vi "PDC_Port.vi"() -> ()   [LabVIEW 2011]
uses:
  <vilib>/Utility/tcp.llb/UDP Multicast Write-Only Open.vi
  <vilib>/Utility/xml.llb/Write to XML File(string).vi
  <vilib>/Utility/xml.llb/Read From XML File(array).vi
  Windows/System32/user32.dll
panel:
  out "output array 5":string[](array[string])
  in  "Analog Params":string[](array[string])
  out "user event out":refnum<user-event>
  in  "Tab Control 3":T1(tab)
  out "Phasor Name":string[](array[string])
  out "Complex Format":cdb[](array[numeric])
  in  "?":i32(listbox)
  out "?":i32(listbox)
  out "?":i32[](listbox)
  out "index of element":i32
  in  "A2":bool[](array[boolean])
  in  "Phasor   Angle":string[](array[string])
  in  "Phasor    Amplitude":string[](array[string])
  out "Row2":i32
  in  "A1":bool[](array[boolean])
  in  "Img":dbl[](array[numeric])
  in  "Real":dbl[](array[numeric])
  in  "Analog Parameters":i32(listbox)
  in  "Digital Parameters":i32(listbox)
  out "Complex":cdb[](array[numeric])
  out "element 2":string
  out "Digital Signal Indicator":bool[][](array[boolean])
  in  "Digital Params":string[](array[string])
  out "element 3":string
  out "Analog Size":i32
  out "Digital Size":i32
  in  "output array":string[](array[string])
  in  "Phasor Item502":string
  in  "Phasor Item402":string
  in  "Phasor Item302":string
  in  "Phasor Item202":string
  in  "Phasor Item102":string
  in  "Phasor Item44":string
  in  "Phasor Item34":string
  in  "Phasor Item24":string
  in  "Phasor Item14":string
  in  "Phasor Item43":string
  in  "Phasor Item33":string
  in  "Phasor Item23":string
  in  "Phasor Item13":string
  in  "Phasor Item42":string
  in  "Phasor Item32":string
  in  "Phasor Item22":string
  in  "Phasor Item12":string
  in  "Phasor Item4":string
  in  "Phasor Item3":string
  in  "Phasor Item2":string
  in  "Phasor Item1":string
  in  "Tab Control 2":T2(tab)
  out "Quitting 2":bool
  in  "Quit 2":bool
  in  "Digital String":string[](array[string])
  in  "Digital Signal":dbl[](array[numeric])
  in  "DFREQ Values":dbl[](array[numeric])
  in  "FREQ Values":dbl[](array[numeric])
  in  "Phasor Values":dbl[](array[numeric])
  in  "Phasor Time":string[](array[string])
  in  "Play Chosen Data":bool
  in  "Load Configuration":bool
  in  "Save Configuration":bool
  out "?":i32[](listbox)
  in  "MA":string
  out "Row of phasor parameter":i32
  out "initialized array":string[](array[string])
  in  "Analog Signal":dbl[](array[numeric])
  out "XML Open File Path":path=path "C:/Users/iitc1/Documents"
  out "XML File Save Path":path
  out "Phasor Index":i32[](array[numeric])
  in  "Display Cluster Output 2":bool
  in  "Display Cluster Output":bool
  out "Phasor_Name":string
  in  "Index of Array of clusters":i32
  out "Rectangular Phasor Values":cdb
  out "Signal Timestamp":string
  out "Phasor Amplitude/Magnitude":dbl
  out "PDC Output Cluster":T3(array[cluster])
  out "FREQ Value":dbl
  out "DFREQ Value":dbl
  in  "OK Button":bool
  in  "Read":bool=TRUE
  in  "Refresh Rate":i64(ring)=200 items=["50 Hz"=20, "20 Hz"=50, "10 Hz"=100, "5 Hz"=200, "2 Hz"=500, "1 Hz"=1000, "Every 2 sec"=2000, "Every 5 sec"=5000, "Every 10 sec"=10000, "Every minute"=60000]
  out "Quitting":bool
  in  "Quit":bool
  out "Status":string
  out "Has New Data?":bool
  out "Connected":bool
  out "Configuration File Received":bool
  out "Buffer Active":bool
  in  "stop":bool
  in  "Phasor_Value_Table":string[](array[string])
  out "concatenated string":string
  in  "Array 2":string[](array[string])
  out "Number of Rows":u32
  out "Listbox":i32(listbox)
  out "x-y*floor(x/y)":i32
  out "x+y":i32
  out "size(s)":i32
  out "element 4":string
  out "stringMessage":string
  out "element":string
  out "Array":string[](array[string])
  out "String":string
  out "Numeric":i32
  out "output array 3":string[](array[string])
  in  "output array 4":string[](array[string])
  in  "Tab Control":T4(tab)
  in  "Save Button":bool
  in  "ID Code":string
  in  "Port":string
  in  "IP Address":string
  in  "output array 2":string[](array[string])
  out "Selected Phasor":string
  in  "?":bool
  in  "PHASORX":string[](array[string])
  out "Row":i32
  out "Row PMU List":i32
  out "bStart":bool
  in  "Local Port":u16=58431
  in  "Send to Port":u16=58432
  in  "TTL":u16=16
  out "error out 2":errorcluster
  in  "Unicast Address":string="192.168.0.101"
  out "Alert Incorrect \nNetwork Info 2":bool
  in  "Local Port 2":u16=58433
  in  "Multicast Address 2":string="234.5.6.7"
  in  "Send to Port 2":u16=58434
  in  "TTL 2":u16=16
  out "error out":errorcluster
  out "Alert Incorrect \nNetwork Info":bool
  out "Waveform Graph":dbl[](graph)
  # "Future Use to Digitals (blinking)."
  # "*Mi  and Ai stand for the Magnitude / Angle of the chosen Phasor, respectively;\n where the index \"i\" is only related to the sequential list of the choice of Data."
  # "Future Use to indicate that frames from the PDC\n are arriving (blinking) with someprotocol flags."
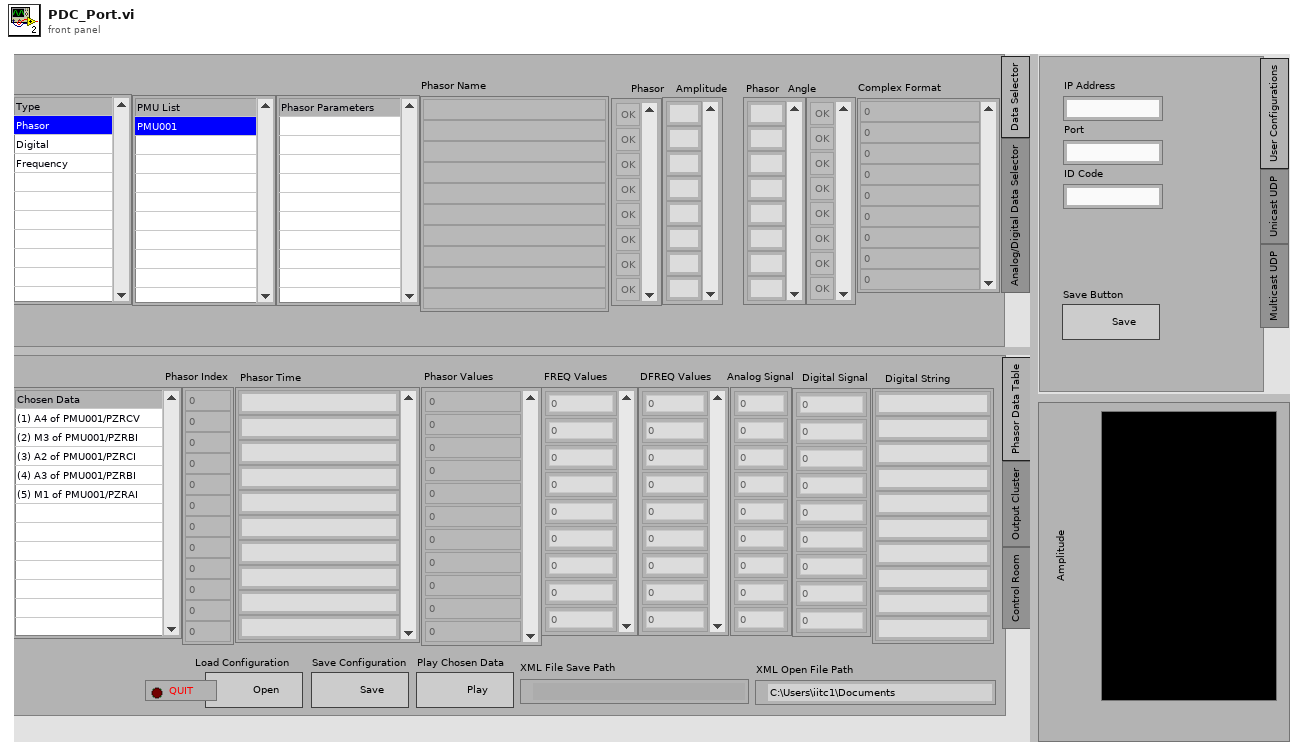
[diagram p1: front panel]
types:
  T1 = enum32{"Data Selector", "Analog/Digital Data Selector"}
  T2 = enum32{"Phasor Data Table", "Output Cluster", "Control Room"}
  T3 = cluster{"Phasor Names":string, "Phasor Timestamp":string, "Phasor Value":dbl, "Rectangular Form":cdb, "DFREQ Value":dbl, "FREQ Value":dbl}[]
  T4 = enum32{"User Configurations", "Unicast UDP", "Multicast UDP"}
  T5 = enum8{"Enabled", "Disabled", "Disabled and Grayed Out"}
  T6 = enum16{"open", "replace", "create", "open or create", "replace or create", "replace or create with confirmation"}
  T7 = cluster{"element":string, "SignalTime":string, "Numeric":dbl, "Numeric":cdb, "Numeric":dbl, "Numeric":dbl}[]
  T8 = cluster{"element":string, "SignalTime":string, "Numeric":dbl, "Numeric":cdb, "Numeric":dbl, "Numeric":dbl}
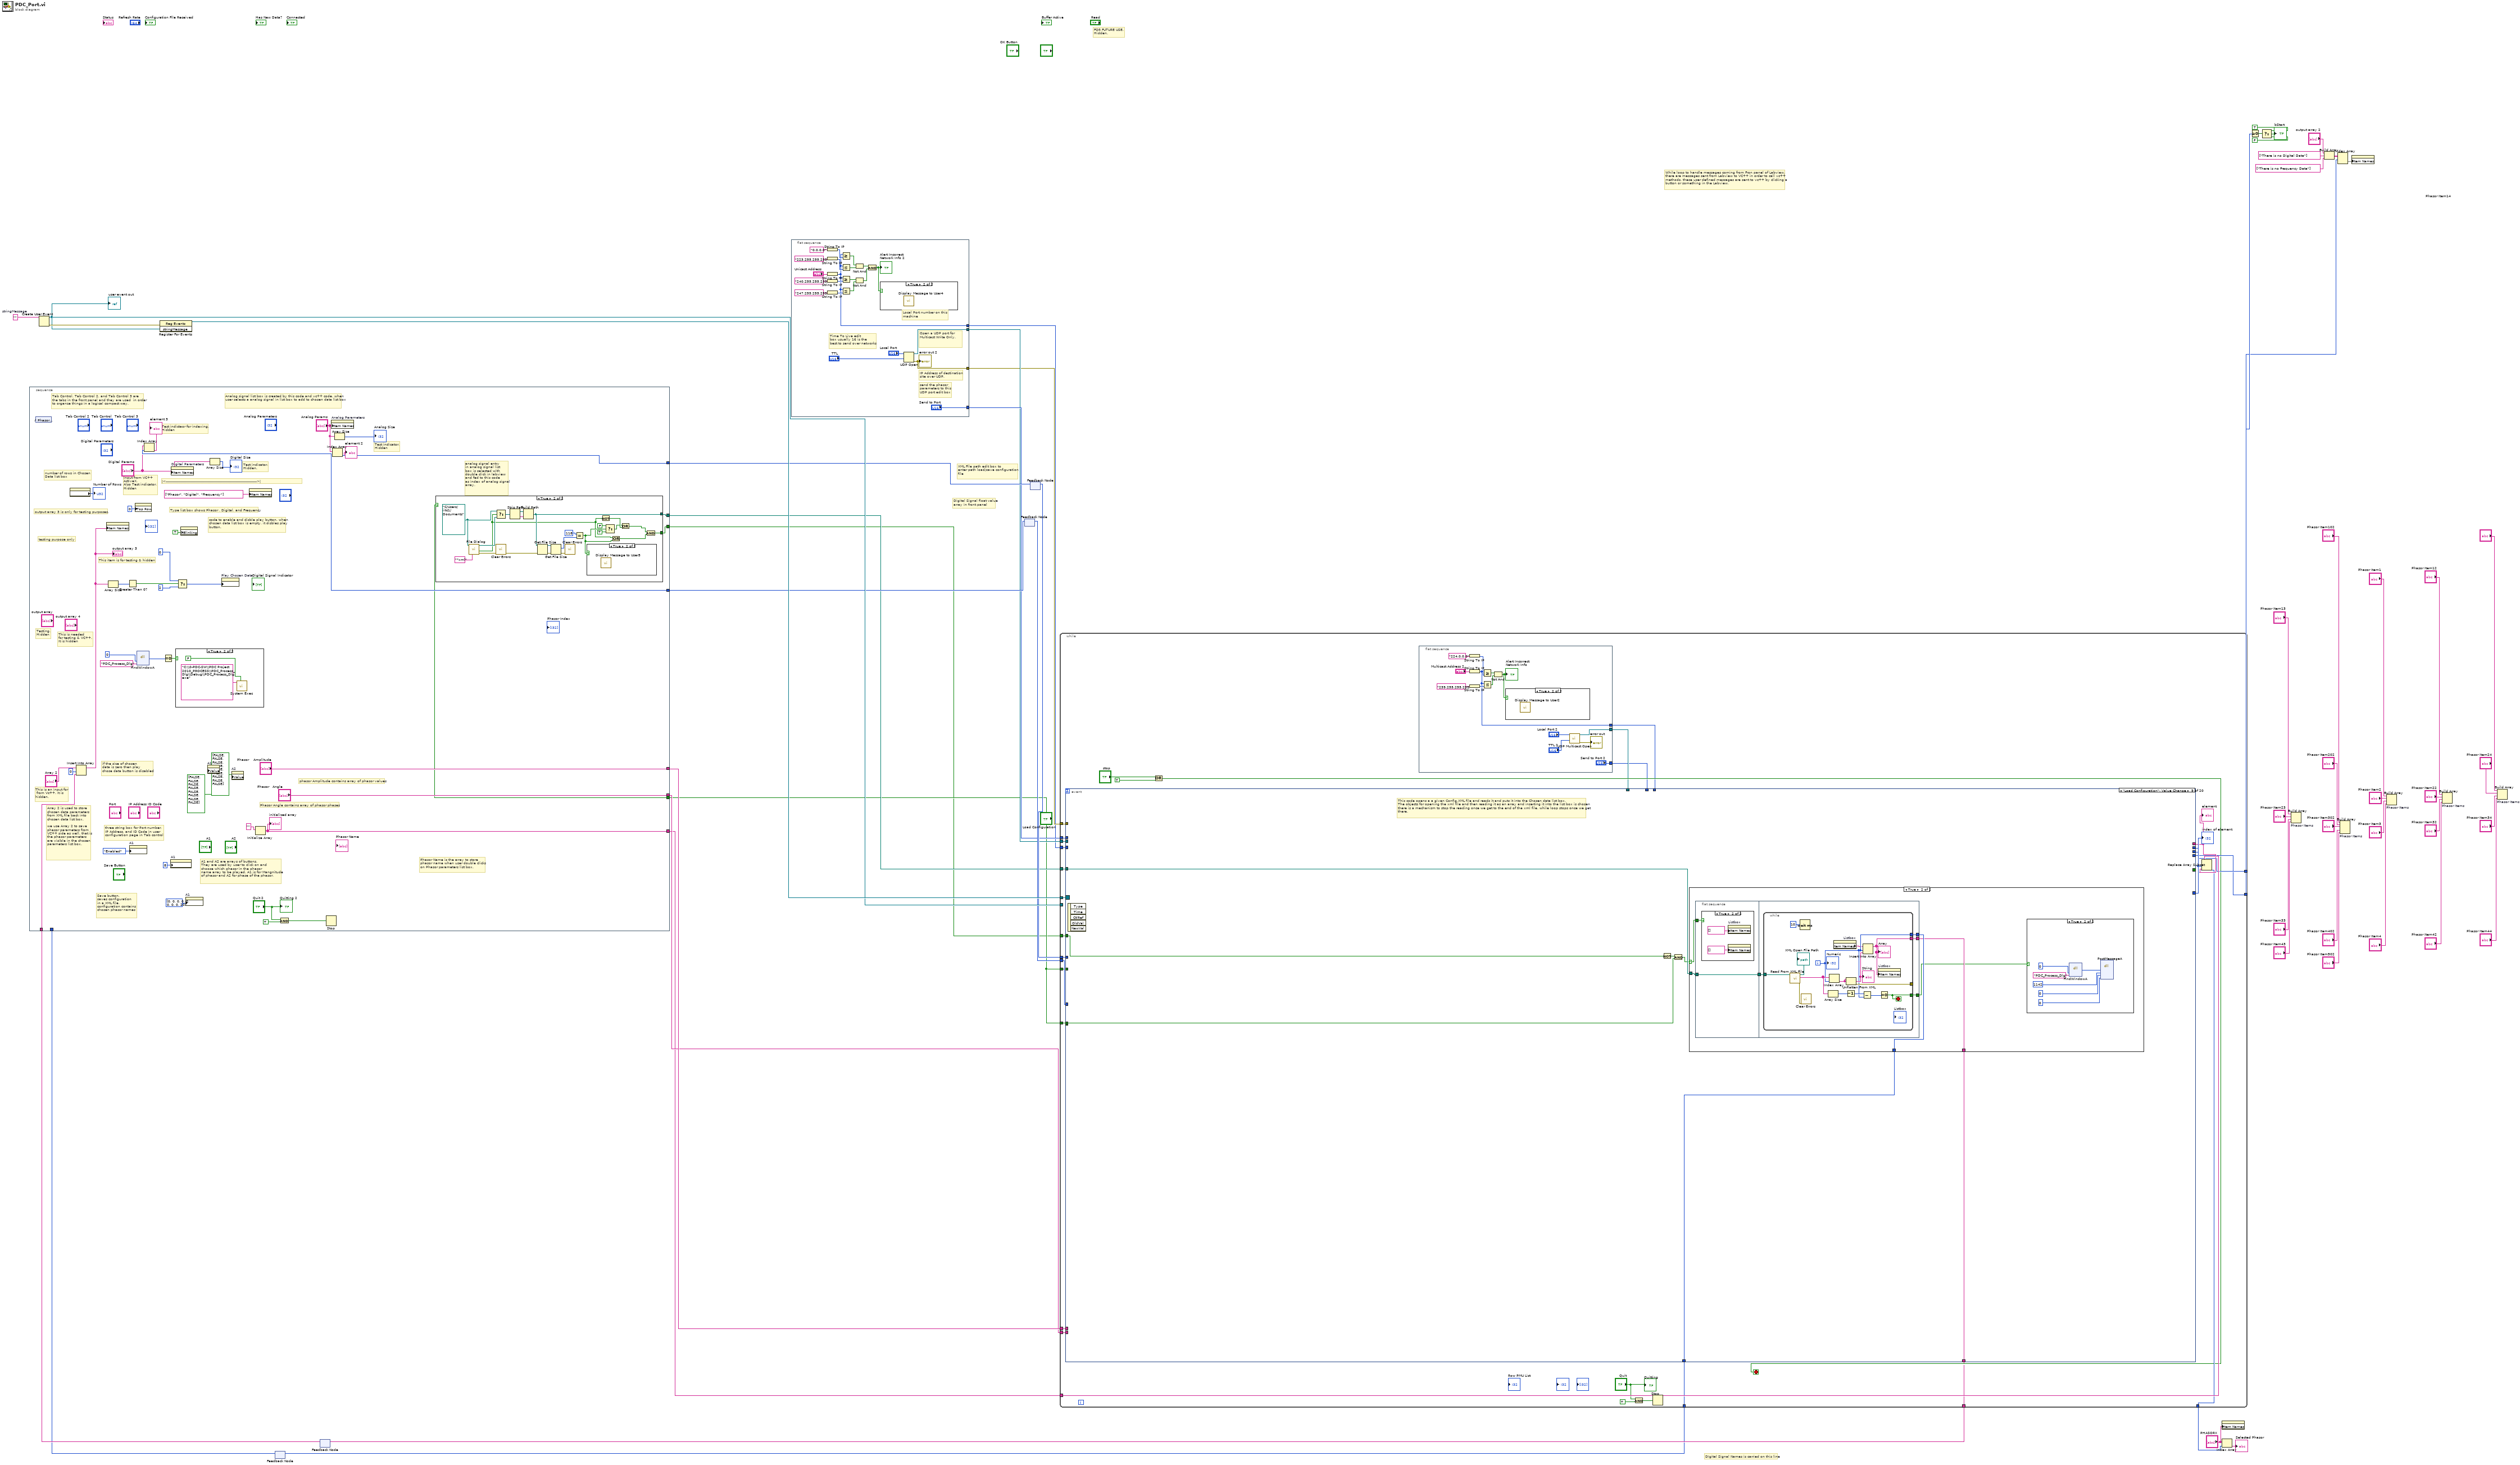
[diagram p0: block diagram]
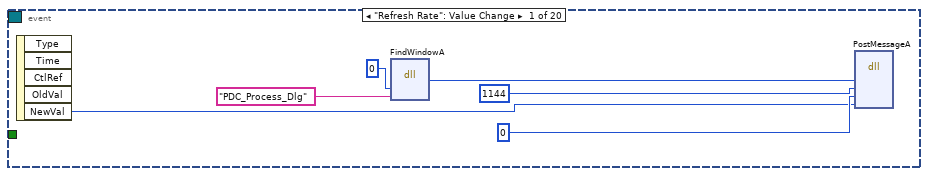
[diagram p4: hidden frame]
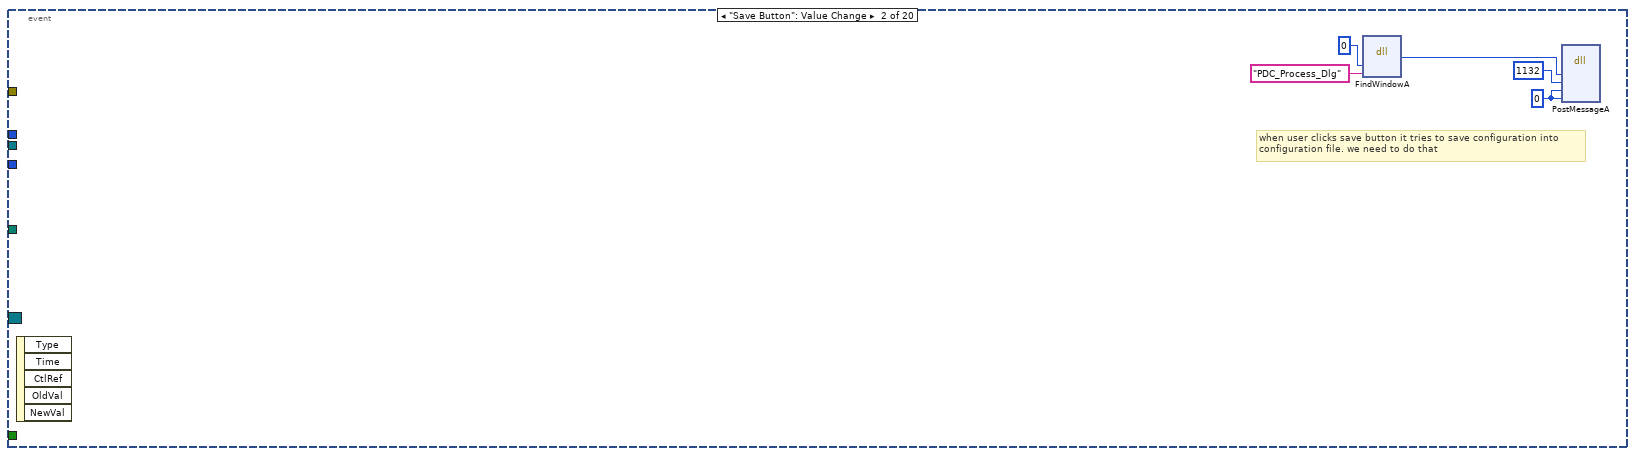
[diagram p5: hidden frame]
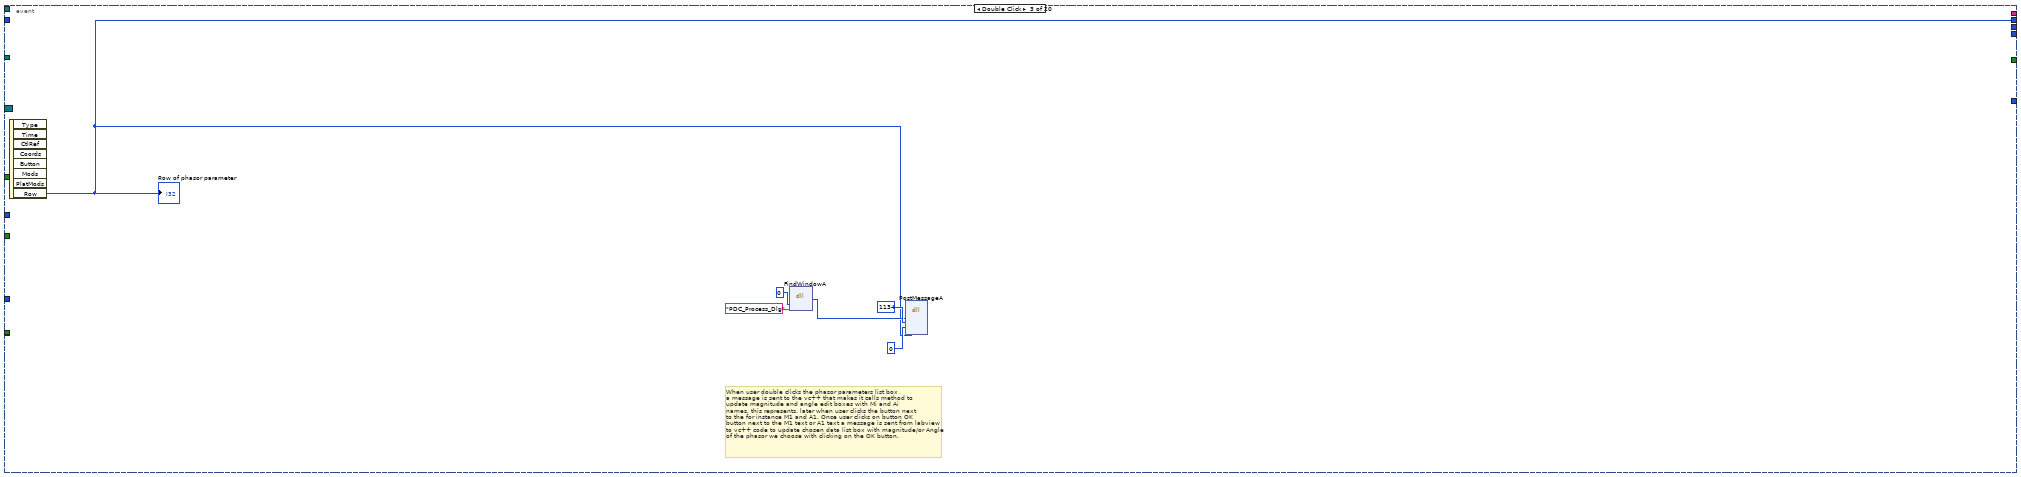
[diagram p6: hidden frame]
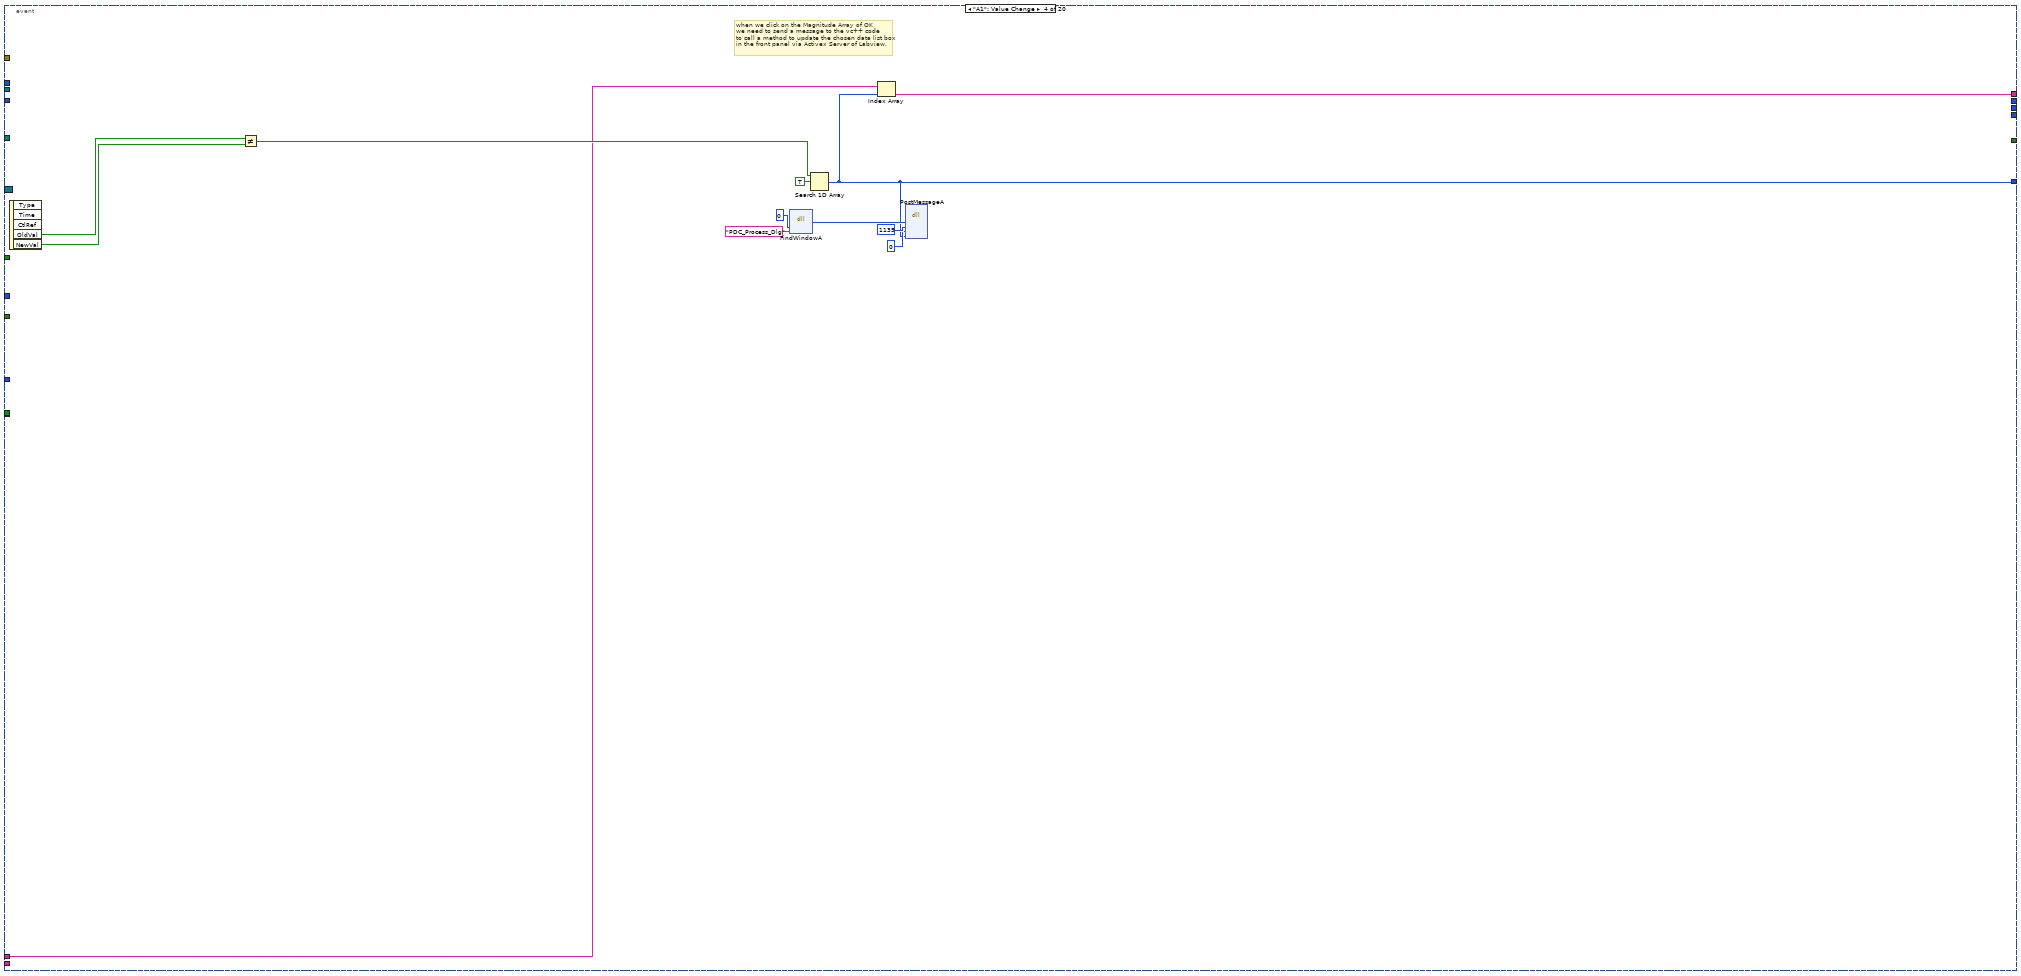
[diagram p7: hidden frame]
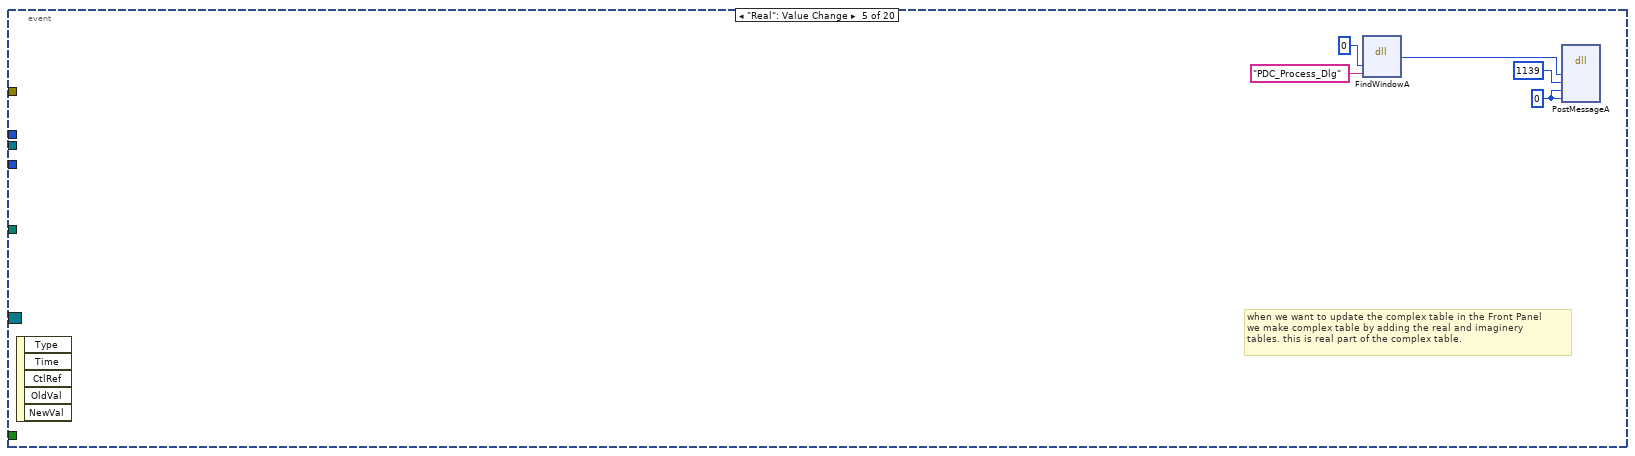
[diagram p8: hidden frame]
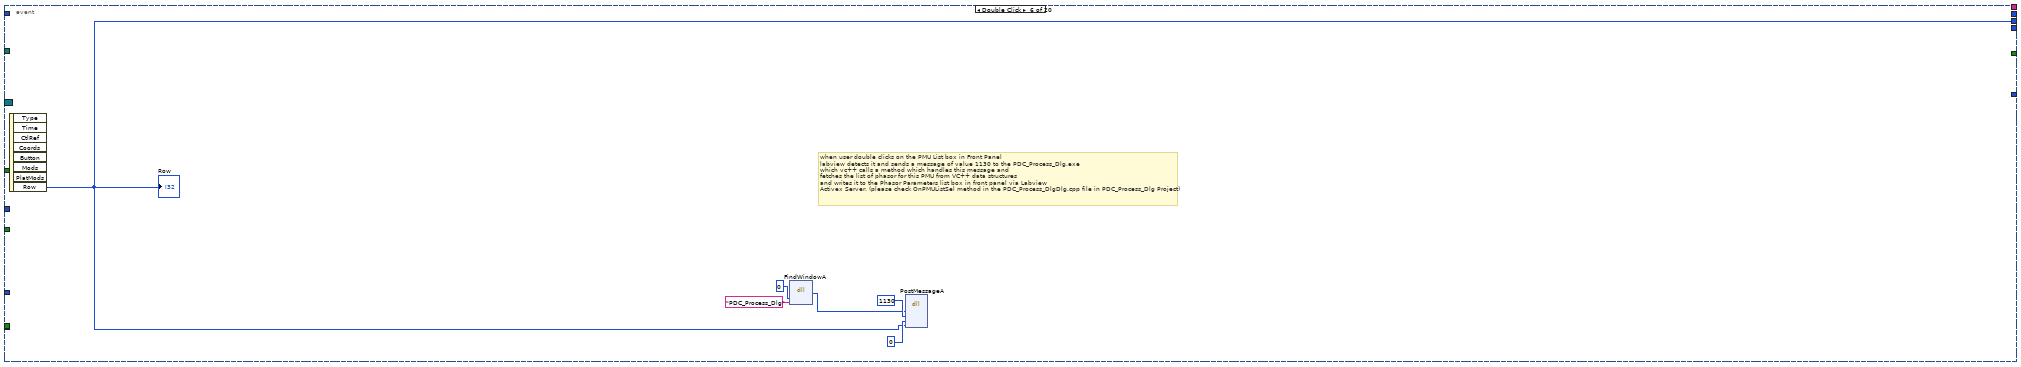
[diagram p9: hidden frame]
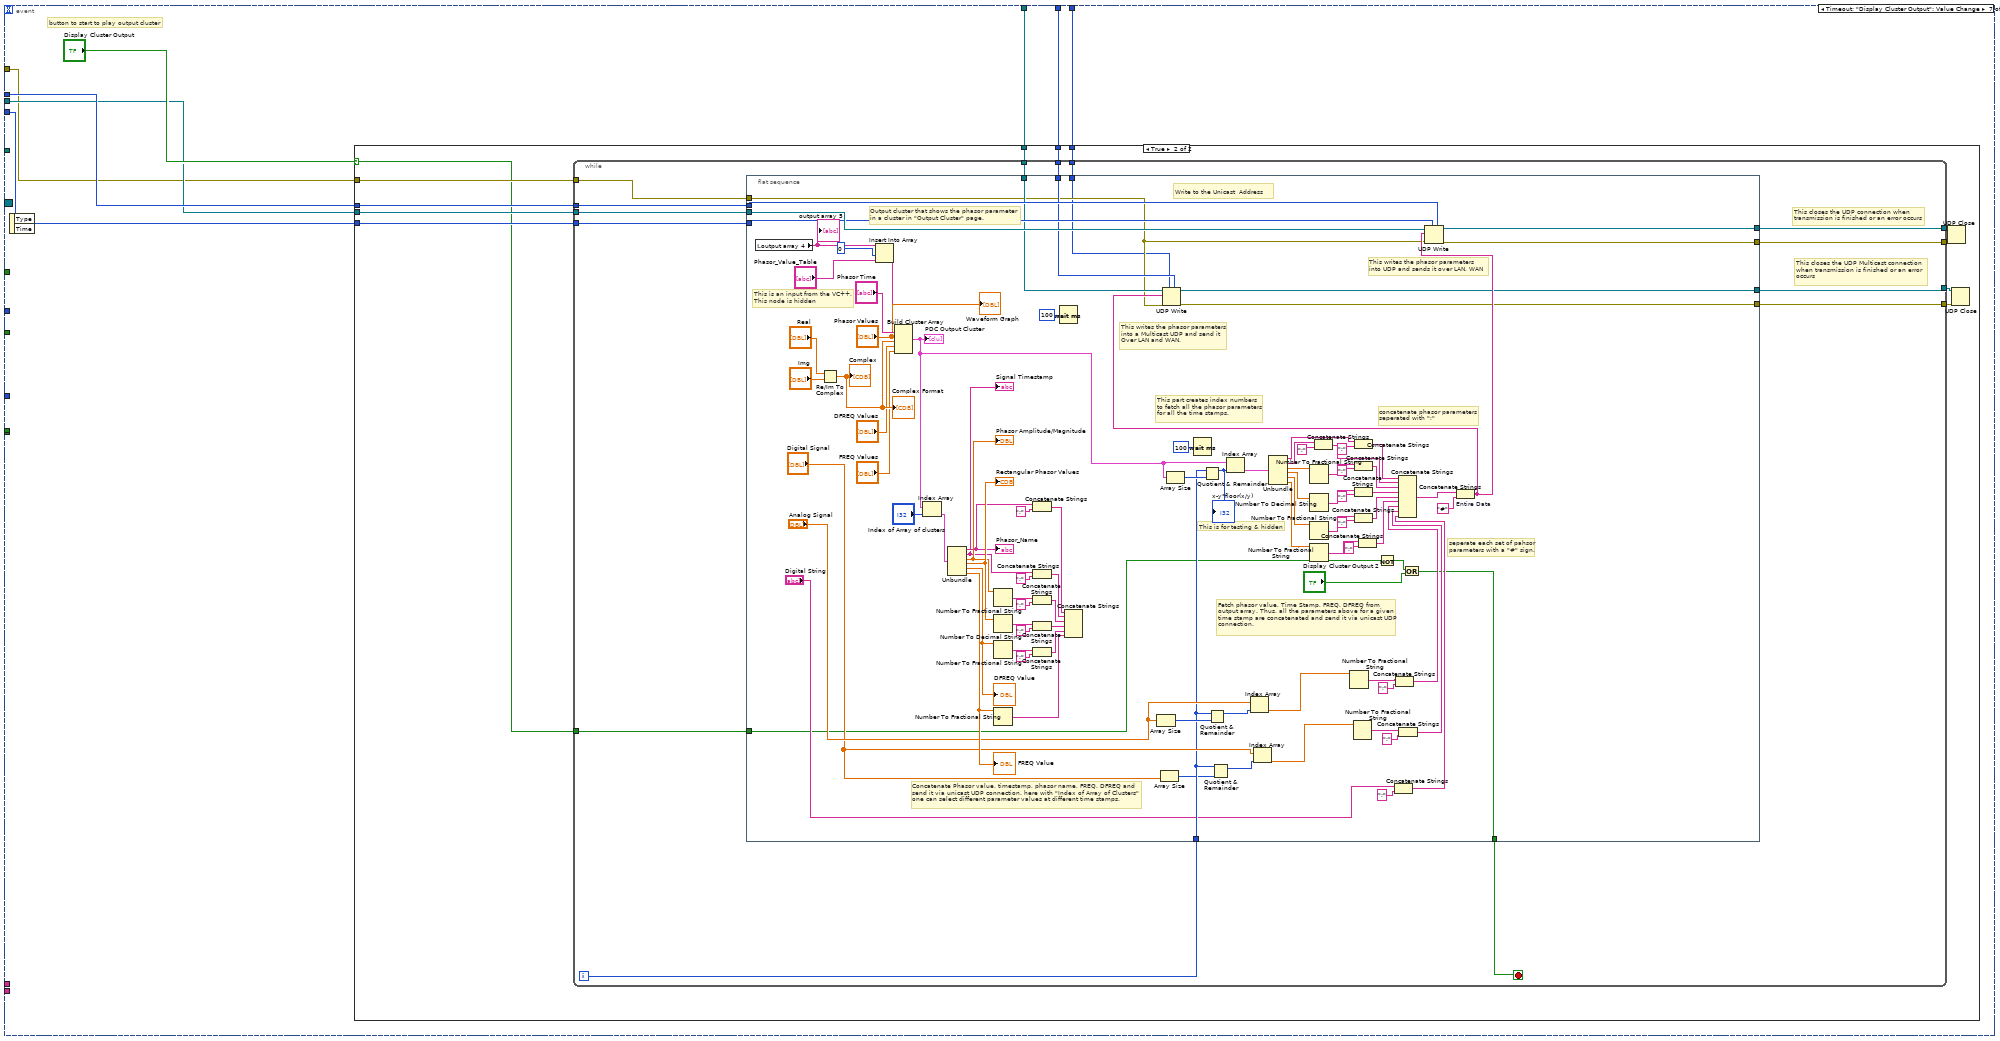
[diagram p10: hidden frame]
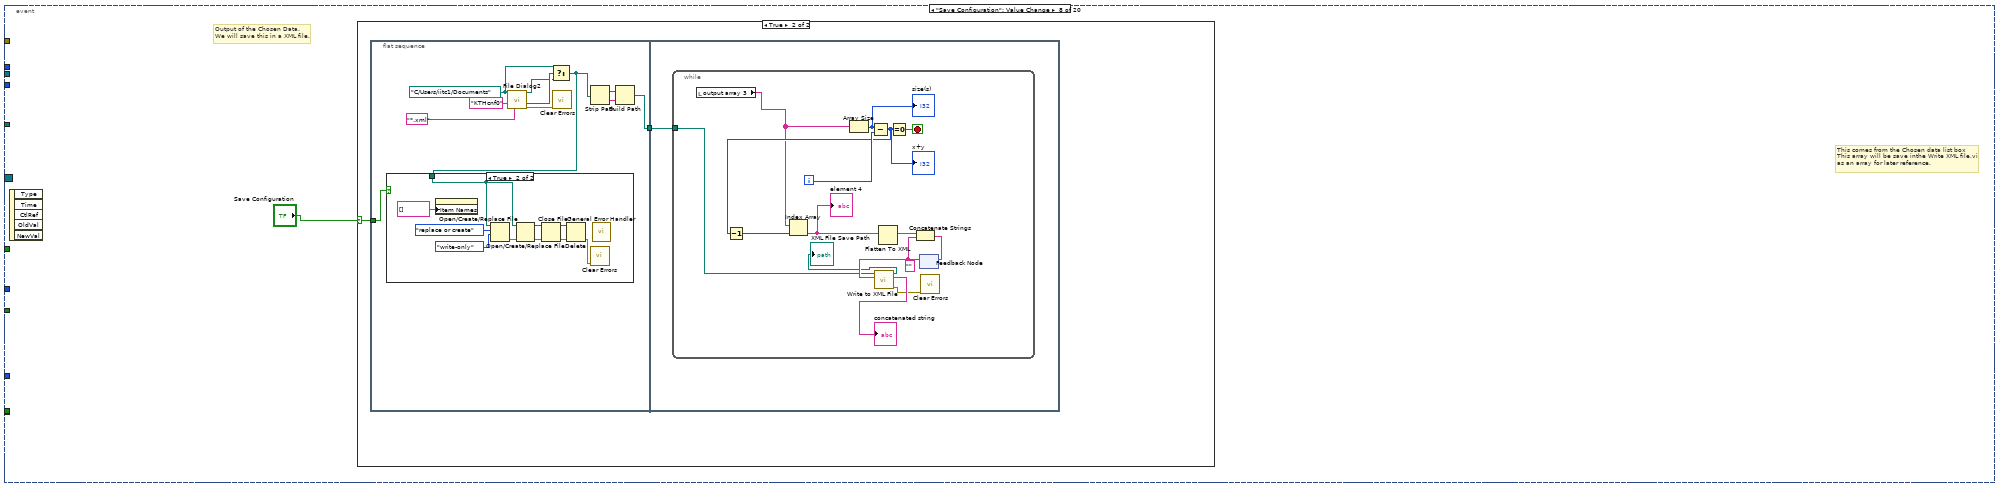
[diagram p12: hidden frame]
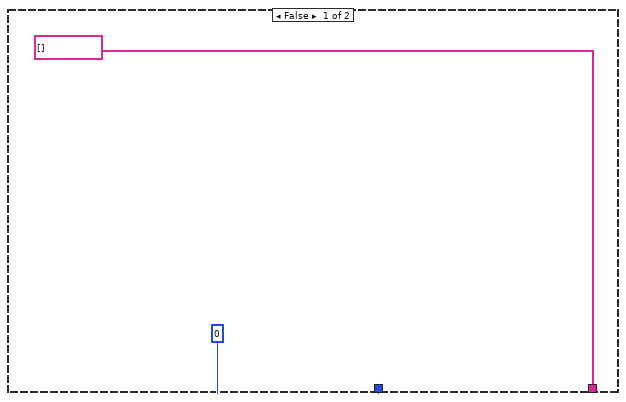
[diagram p15: hidden frame]
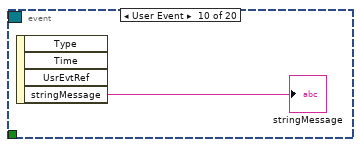
[diagram p18: hidden frame]
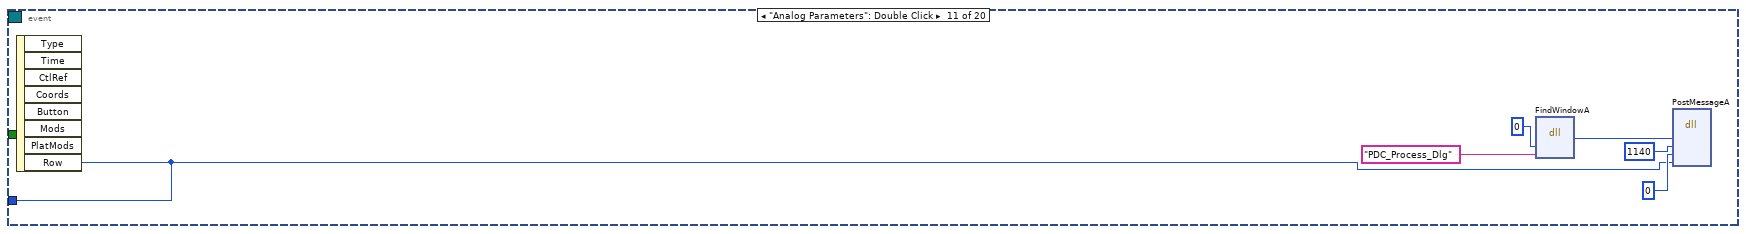
[diagram p19: hidden frame]
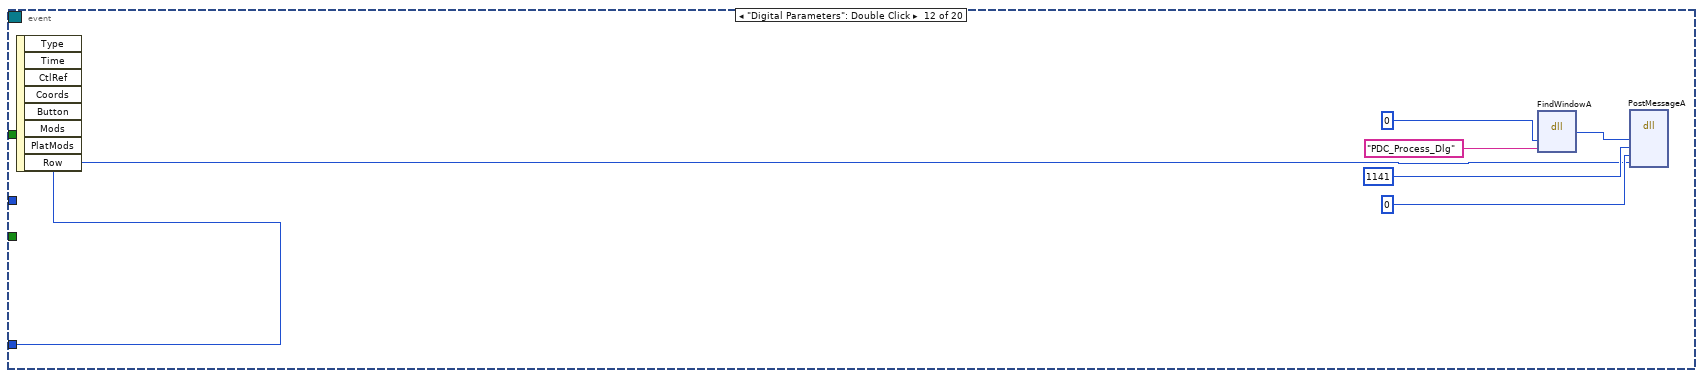
[diagram p20: hidden frame]
diagram:
  w18 = ""  # stringMessage
  # "FOR FUTURE USE.\nHidden."
  # "DIgital Signal Names is carried on this line"
  # "XML File path edit box to \nenter path load/save configuration\nfile"
  # "Digital Signal float value\narray in front panel"
  # "While loop to handle messages coming from Fron panel of Labview. \nthere are messages sent from Labview to VC++ in order to call vc++\nmethods. these user defined messages are sent to vc++ by clicking a \nbutton or something in the Labview."
  n1 = Create User Event(user event datatype=w18) -> (user event=w16:refnum<user-event>, error out=w19:errorcluster)  [unwired: 1 in]
  "user event out" <- w16
  n2 = register-events(error in=w19, w16) -> (reference out=w17:refnum<event-registration>)  [unwired: 1 in, 1 out]
  n3 = feedback #1() -> (w6:i32)  [unwired: 1 in]
  n4 = feedback #2() -> (w8:string[])  [unwired: 1 in]
  n5 = flat-sequence {
    tunnel: ["Send to Port"] -> w11
    tunnel: [w76] -> w10
    tunnel: [w75] -> w5
    tunnel: [w63] -> w4
    frame #0 {
      # "Local Port number on this\nmachine"
      # "Time To Live edit\nbox usually 16 is the\nbest to send over networks"
      # "IP Address of destination\nsite over UDP."
      # "send the phasor\nparameters to this\nUDP port edit box"
      # "Open a UDP port for Multicast Write Only."
      n6 = String To IP(1:"0.0.0.0" ("x")) -> (0:w72:u32)
      n7 = String To IP(1:"223.255.255.255" ("x")) -> (0:w71:u32)
      n8 = String To IP(1:"Unicast Address") -> (0:w63:u32)
      n9 = String To IP(1:"240.255.255.255" ("x")) -> (0:w67:u32)
      n10 = String To IP(1:"247.255.255.255" ("x")) -> (0:w66:u32)
      n11 = Greater Or Equal?(x=w63, y=w72) -> (x >= y?=w74:bool)
      n12 = Less Or Equal?(x=w63, y=w71) -> (x <= y?=w73:bool)
      n13 = Greater Or Equal?(x=w63, y=w67) -> (x >= y?=w62:bool)
      n14 = Less Or Equal?(x=w63, y=w66) -> (x <= y?=w61:bool)
      n15 = Not And(1:w73, 2:w74) -> (0:w60:bool)
      n16 = Not And(1:w61, 2:w62) -> (0:w59:bool)
      n17 = And(x=w60, y=w59) -> (x .and. y?=w58:bool)
      "Alert Incorrect \nNetwork Info 2" <- w58
      n18 = case shown="True" w58 {
        frame False {
        }
        frame True {
          n19 = call "Display Message to User4"() -> ()  [unwired: 10 in, 2 out]
        }
      }
      n20 = UDP Open(9:"TTL", 11:"Local Port") -> (port=w76:refnum<k16>, 0:w75:errorcluster)  [unwired: 3 in, 1 out]
      "error out 2" <- w75
    }
  }
  n21 = feedback #3() -> (w12:i32)  [unwired: 1 in]
  n22 = feedback #4() -> (w14:i32)  [unwired: 1 in]
  n23 = stacked-sequence {
    tunnel: ["Phasor    Amplitude"] -> w57
    tunnel: ["Phasor   Angle"] -> w56
    tunnel: [w119] -> w55
    tunnel: w14 -> [w111]
    tunnel: w12 -> [w109]
    tunnel: w8 -> [w93]
    tunnel: [w104] -> _
    tunnel: w6 -> [w104]
    tunnel: [w92] -> w3
    tunnel: "Load Configuration" -> [w91]
    tunnel: [w90] -> w1
    frame #0 {
      # "Test indictaor for indexing.\nHidden"
      # "Input from VC++\nActiveX. \nAlso Test indicator.\nHidden"
      # "Test indicator.\nHidden."
      # "Test indicator.\nHidden"
      # "Testing.\nHidden"
      # "This is needed\nfor testing & VC++.\nIt is hidden"
      # "This is an input for\n from Vc++. It is\nhidden."
      # "This item is for testing & hidden"
      # "if the size of chosen\ndata is zero then play\nchose data button is disabled"
      # "output array 3 is only for testing purposes."
      # "testing purpose only"
      # "Array 2 is used to store\nchosen data parameters\nfrom XML file back into\nchosen data list box.\n\nwe use Array 2 to save \nphasor parameters from\nVC++ side as well. that is\nthe phasor parameters \nare visible in the chosen\nparameters list box."
      # "Phasor Angle contains array of phasor phases"
      # "phasor Amplitude contains array of phasor values"
      # "Save button, \nsaves configuration\nin a XML file. \nconfiguration contains\nchosen phasor names"
      # "A1 and A2 are arrays of buttons.\nThey are used by user to click on and\nchoose which phasor in the phasor \nname array to be played. A1 is for Mangnitude\nof phasor and A2 for phase of the phasor."
      # "Phasor Name is the array to store\nphasor name when user double clicks\non Phasor parameters list box."
      # "three string box for Port number,\nIP Address, and ID Code in user\nconfiguration page in Tab control"
      # "code to enable and disble play button. when\nchosen data list box is empty, it disbles play\nbutton."
      # "analog signal entry\nin analog signal list\nbox is selected with\ndouble click in labview\nand fed to this code\nas index of analog signal\narray."
      # "Analog signal list box is created by this code and vc++ code. when\nuser selects a analog signal in list box to add to chosen data list box"
      # "|<--------------------------------------------------------------------------------->|"
      # "Type list box shows Phasor , Digital, and Frequency"
      # "number of rows in Chosen\nData list box"
      # "Tab Control, Tab Control 2, and Tab Control 3 are\nthe tabs in the front panel and they are used  in order\nto organze things in a logical compact way."
      n24 = control-ref of="Phasor   Angle"() -> ()  [unwired: 1 out]
      n25 = property class="LstBox (strict)"() -> ("Number of Rows"=→"Number of Rows":u32)  [unwired: 2 in, 2 out]
      n26 = Insert Into Array(array="Array 2", index=0, new element=w93) -> (w99:string[])
      "output array 3" <- w99
      n27 = property class="LstBox (strict)"("Item Names"=w99) -> ()  [unwired: 2 in, 2 out]
      n28 = Array Size(array=w99) -> (size(s)=w102:i32)
      n29 = Greater Than 0?(x=w102) -> (x > 0?=w116:bool)
      n30 = property on="A1" class="Arr (strict)"("DisabledEnum"=T5."Enabled" ("Disabled")) -> ()  [unwired: 2 in, 2 out]
      n31 = property class="LstBox (strict)"("Top Row"=0) -> ()  [unwired: 2 in, 2 out]
      n32 = dll-call lib="C:/Windows/System32/user32.dll" fn="FindWindowA"("lpszClassName"=0, "lpszWindowName"="PDC_Process_Dlg") -> ("return type"=w81:i32)  [unwired: 5 in, 2 out]
      n33 = Index Array(array="Digital Params", index=w109) -> (element=→"element 3":string)
      n34 = Equal To 0?(x=w81) -> (x = 0?=w80:bool)
      n35 = property on="A1" class="Arr (strict)"("Number of Rows"=u32 8) -> ()  [unwired: 2 in, 2 out]
      n36 = property on="Digital Parameters" class="LstBox (strict)"("Item Names"="Digital Params") -> ()  [unwired: 2 in, 2 out]
      n37 = case shown="True" w80 {
        frame False {
        }
        frame True {
          n38 = call <vilib>:"System Exec.vi"("wait until completion? (T)"=FALSE, "command line"="C:\\0-PDC-SW\\PDC Project 2010_PROCESS\\PDC_Process_Dlg\\Debug\\PDC_Process_Dlg.exe") -> ()  [unwired: 6 in, 4 out]
        }
      }
      n39 = Select(t=u32 0, s=w116, f=u32 2) -> (s? t:f=w100:u32)
      n40 = property class="LstBox (strict)"("Blinking"=TRUE) -> ()  [unwired: 2 in, 2 out]
      n41 = property on="A1" class="Arr (strict)"("Selection Start []"=u32[] [0, 0, 0, 0, 0, 0, 0, 0, 20] ("Selection Start[]")) -> ()  [unwired: 2 in, 2 out]
      n42 = property on="A1" class="Arr (strict)"("Value"=bool[] [FALSE, FALSE, FALSE, FALSE, FALSE, FALSE, FALSE, FALSE] ("A1")) -> ()  [unwired: 2 in, 2 out]
      n43 = Array Size(array="Digital Params") -> (size(s)=→"Digital Size":i32)
      n44 = property on="Play Chosen Data" class="Bool"("DisabledEnum"=w100) -> ()  [unwired: 2 in, 2 out]
      n45 = property on="A2" class="Arr (strict)"("Value"=bool[] [FALSE, FALSE, FALSE, FALSE, FALSE, FALSE, FALSE, FALSE, FALSE] ("A2")) -> ()  [unwired: 2 in, 2 out]
      n46 = property class="LstBox (strict)"("Item Names"=string[] ["Phasor", "Digital", "Frequency"]) -> ()  [unwired: 2 in, 2 out]
      n47 = Initialize Array("" ("element")) -> (w119:string[])  [unwired: 1 in]
      "initialized array" <- w119
      n48 = And(x="Quit 2", y=TRUE) -> (x .and. y?=w96:bool)
      n49 = Stop(stop? (T)=w96) -> ()
      n50 = property on="Analog Parameters" class="LstBox (strict)"("Item Names"="Analog Params") -> ()  [unwired: 2 in, 2 out]
      n51 = Index Array(array="Analog Params", index=w111) -> (element=→"element 2":string)
      n52 = Array Size(array="Analog Params") -> (size(s)=→"Analog Size":i32)
      n53 = case shown="True" w91 {
        tunnel: [_ w133] -> w92
        tunnel: [_ w125] -> w90
        frame False {
        }
        frame True {
          w142 = path "C:/Users/iitc1/Documents" ("start path")
          n54 = call "File Dialog"("start path"=w142, "pattern (all files)"="*xml") -> ("selected path"=w134:path, "cancelled"=w126:bool, "error out"=w140:errorcluster)  [unwired: 10 in, 1 out]
          n55 = Select(t=w142, s=w126, f=w134) -> (s? t:f=w141:path)
          n56 = call <vilib>:"Clear Errors.vi"("error in (no error)"=w140) -> ("error out"=w139:errorcluster)  [unwired: 6 in]
          n57 = Strip Path(path=w141) -> (stripped path=w145:path, name=w144:string)
          n58 = Build Path(base path=w145, name or relative path=w144) -> (appended path=w133:path)
          n59 = Get File Size(file=w133, error in=w139) -> (refnum out=w138:refnum<file>, 0:w135:errorcluster)  [unwired: 1 out]
          n60 = Get File Size(file=w138, error in=w135) -> (size (in bytes)=w137:i64, 0:w132:errorcluster)  [unwired: 1 out]
          n61 = call <vilib>:"Clear Errors.vi"("error in (no error)"=w132) -> ()  [unwired: 6 in, 1 out]
          n62 = Equal?(x=i64 118, y=w137) -> (x = y?=w127:bool)
          n63 = case shown="True" w127 {
            frame False {
            }
            frame True {
              n64 = call "Display Message to User3"() -> ()  [unwired: 10 in, 2 out]
            }
          }
          n65 = Not(x=w126) -> (.not. x?=w129:bool)
          n66 = Select(t=FALSE, s=w127, f=TRUE) -> (s? t:f=w128:bool)
          n67 = Or(x=w126, y=w127) -> (x .or. y?=w124:bool)
          n68 = Or(x=w128, y=w129) -> (x .or. y?=w123:bool)
          n69 = And(x=w123, y=w124) -> (x .and. y?=w125:bool)
        }
      }
      "Quitting 2" <- "Quit 2"
    }
  }
  n70 = while {
    tunnel: w57 -> [w175]
    tunnel: w56 -> [w174]
    tunnel: w55 -> [w173]
    tunnel: [w170] -> w29
    tunnel: [w169] -> w28
    tunnel: [w168] -> w21
    tunnel: w16 -> [_]
    tunnel: w17 -> [w164]
    tunnel: [w163] -> w15
    tunnel: [w162] -> w13
    tunnel: w11 -> [w161]
    tunnel: w4 -> [w160]
    tunnel: w10 -> [w159]
    tunnel: w5 -> [w158]
    tunnel: w3 -> [w157]
    tunnel: [w156] -> w9
    tunnel: [w155] -> w7
    tunnel: "Load Configuration" -> [w154]
    tunnel: "Load Configuration" -> [w153]
    tunnel: w1 -> [w146]
    stop <- w165 stop-if-true
    n71 = event shown="[8] \"Load Configuration\": Value Change" {
      selector: w164 -> [_ _ _ _ _ _ _ _ _ _ _ _ _ _ _ _ _ _ _ _]
      dyn-events: _ -> [_ _ _ _ _ _ _ _ _ _ _ _ _ _ _ _ _ _ _ _]
      timeout: _ -> [_ _ _ _ _ _ _ _ _ _ _ _ _ _ _ _ _ _ _ _]
      tunnel: [_ _ _ w214 _ _ _ _ _ _ _ _ _ _ _ _ _ _ w511 _] -> w171
      tunnel: [_ _ _ w207 _ _ _ _ _ _ _ _ _ _ _ _ _ _ w503 _] -> w172
      tunnel: w175 -> [_ _ _ w213 _ _ _ _ _ _ _ _ _ _ _ _ _ _ _ _]
      tunnel: w174 -> [_ _ _ _ _ _ _ _ _ _ _ _ _ _ _ _ _ _ w509 _]
      tunnel: [_ _ _ _ _ w224 _ _ _ _ _ _ _ _ _ _ _ _ _ _] -> w170
      tunnel: [_ _ _ _ _ _ _ _ _ _ _ _ w457 _ _ _ _ _ _ _] -> w169
      tunnel: [_ _ w201 _ _ _ _ _ _ _ _ _ _ _ _ _ _ _ _ _] -> w168
      tunnel: [_ _ _ _ _ _ _ _ _ _ _ _ _ _ w469 _ _ _ _ _] -> _
      tunnel: [_ _ _ _ _ _ _ _ _ _ w445 _ _ _ _ _ _ _ _ _] -> w163
      tunnel: [_ _ _ _ _ _ _ _ _ _ _ w451 _ _ _ _ _ _ _ _] -> w162
      tunnel: w161 -> [_ _ _ _ _ _ w236 _ _ _ _ _ _ _ _ _ _ _ _ _]
      tunnel: w160 -> [_ _ _ _ _ _ w235 _ _ _ _ _ _ _ _ _ _ _ _ _]
      tunnel: w159 -> [_ _ _ _ _ _ w234 _ _ _ _ _ _ _ _ _ _ _ _ _]
      tunnel: w158 -> [_ _ _ _ _ _ w233 _ _ _ _ _ _ _ _ _ _ _ _ _]
      tunnel: w157 -> [_ _ _ _ _ _ _ _ w404 _ _ _ _ _ _ _ _ _ _ _]
      tunnel: [_ _ _ _ _ _ _ _ w405 _ _ _ _ _ _ _ _ _ _ _] -> w156
      tunnel: [_ _ _ _ _ _ _ _ w406 _ _ _ _ _ _ _ _ _ _ _] -> w155
      tunnel: [_ _ _ _ _ _ _ _ w403 _ _ _ _ _ _ _ _ _ _ _] -> _
      tunnel: w154 -> [_ _ _ _ _ _ _ _ w403 _ _ _ _ _ _ _ _ _ _ _]
      tunnel: w153 -> [_ _ _ _ _ _ _ _ _ _ _ _ _ _ _ _ w495 _ _ _]
      tunnel: w147 -> [_ _ _ _ _ _ w232 _ _ _ _ _ _ _ _ _ _ _ _ _]
      tunnel: w148 -> [_ _ _ _ _ _ w231 _ _ _ _ _ _ _ _ _ _ _ _ _]
      tunnel: w149 -> [_ _ _ _ _ _ w230 _ _ _ _ _ _ _ _ _ _ _ _ _]
      tunnel: w146 -> [_ _ _ _ _ _ _ _ w401 _ _ _ _ _ _ _ _ _ _ _]
      event "Refresh Rate": Value Change {
        n72 = event-data() -> ("NewVal"=w190:i64)  [unwired: 1 in, 4 out]
        n73 = dll-call lib="C:/Windows/System32/user32.dll" fn="FindWindowA"("lpszClassName"=0, "lpszWindowName"="PDC_Process_Dlg" ("lpszWindowName 2")) -> ("return type"=w192:i32)  [unwired: 5 in, 2 out]
        n74 = dll-call lib="C:/Windows/System32/user32.dll" fn="PostMessageA" label="SendMessageA"("hWnd"=w192, "uMsg"=1144, "wParam"=0, "lParam"=w190) -> ()  [unwired: 8 in, 2 out]
      }
      event "Save Button": Value Change {
        w196 = 0 ("wParam")
        # "when user clicks save button it tries to save configuration into\nconfiguration file. we need to do that"
        n75 = event-data() -> ()  [unwired: 1 in, 5 out]
        n76 = dll-call lib="C:/Windows/System32/user32.dll" fn="FindWindowA"("lpszClassName"=0, "lpszWindowName"="PDC_Process_Dlg" ("lpszWindowName 3")) -> ("return type"=w197:i32)  [unwired: 5 in, 2 out]
        n77 = dll-call lib="C:/Windows/System32/user32.dll" fn="PostMessageA" label="SendMessageA"("hWnd"=w197, "uMsg"=1132, "wParam"=w196, "lParam"=w196) -> ()  [unwired: 8 in, 2 out]
      }
      event Double Click {
        # "When user double clicks the phasor parameters list box\na message is sent to the vc++ that makes it calls method to \nupdate magnitude and angle edit boxes with Mi and Ai \nnames. this represents. later when user clicks the button next\nto the for instance M1 and A1. Once user clicks on button OK \nbutton next to the M1 text or A1 text a message is sent from labview \nto vc++ code to update chosen data list box with magnitude/or Angle\nof the phasor we choose with clicking on the OK button."
        n78 = event-data() -> ("Row"=w201:i32)  [unwired: 1 in, 7 out]
        "Row of phasor parameter" <- w201
        n79 = dll-call lib="C:/Windows/System32/user32.dll" fn="FindWindowA"("lpszClassName"=0, "lpszWindowName"="PDC_Process_Dlg" ("lpszWindowName 2")) -> ("return type"=w203:i32)  [unwired: 5 in, 2 out]
        n80 = dll-call lib="C:/Windows/System32/user32.dll" fn="PostMessageA" label="SendMessageA"("hWnd"=w203, "uMsg"=1134, "wParam"=0, "lParam"=w201) -> ()  [unwired: 8 in, 2 out]
      }
      event "A1": Value Change {
        # "when we click on the Magnitude Array of OK\nwe need to send a message to the vc++ code\nto call a method to update the chosen data list box\nin the front panel via Activex Server of Labview."
        n81 = event-data() -> ("OldVal"=w218:bool[], "NewVal"=w217:bool[])  [unwired: 1 in, 3 out]
        n82 = Not Equal?(x=w218, y=w217) -> (x != y?=w216:bool[])
        n83 = dll-call lib="C:/Windows/System32/user32.dll" fn="FindWindowA"("lpszClassName"=0, "lpszWindowName"="PDC_Process_Dlg" ("lpszWindowName 2")) -> ("return type"=w209:i32)  [unwired: 5 in, 2 out]
        n84 = Search 1D Array(1D array=w216, element=TRUE) -> (index of element=w207:i32)  [unwired: 1 in]
        n85 = Index Array(array=w213, index=w207) -> (element=w214:string)
        n86 = dll-call lib="C:/Windows/System32/user32.dll" fn="PostMessageA" label="SendMessageA"("hWnd"=w209, "uMsg"=1135, "wParam"=0, "lParam"=w207) -> ()  [unwired: 8 in, 2 out]
      }
      event "Real": Value Change {
        w219 = 0 ("wParam")
        # "when we want to update the complex table in the Front Panel\nwe make complex table by adding the real and imaginery\ntables. this is real part of the complex table."
        n87 = event-data() -> ()  [unwired: 1 in, 5 out]
        n88 = dll-call lib="C:/Windows/System32/user32.dll" fn="FindWindowA"("lpszClassName"=0, "lpszWindowName"="PDC_Process_Dlg" ("lpszWindowName 2")) -> ("return type"=w220:i32)  [unwired: 5 in, 2 out]
        n89 = dll-call lib="C:/Windows/System32/user32.dll" fn="PostMessageA" label="SendMessageA"("hWnd"=w220, "uMsg"=1139, "wParam"=w219, "lParam"=w219) -> ()  [unwired: 8 in, 2 out]
      }
      event Double Click {
        # "when user double clicks on the PMU List box in Front Panel\nlabview detects it and sends a message of value 1130 to the PDC_Process_Dlg.exe\nwhich vc++ calls a method which handles this message and\nfetches the list of phasor for this PMU from VC++ data structures\nand writes it to the Phasor Parameters list box in front panel via Labview\nActivex Server. (please check OnPMUListSel method in the PDC_Process_DlgDlg.cpp file in PDC_Process_Dlg Project)"
        n90 = event-data() -> ("Row"=w224:i32)  [unwired: 1 in, 7 out]
        "Row" <- w224
        n91 = dll-call lib="C:/Windows/System32/user32.dll" fn="FindWindowA"("lpszClassName"=0, "lpszWindowName"="PDC_Process_Dlg" ("lpszWindowName 2")) -> ("return type"=w226:i32)  [unwired: 5 in, 2 out]
        n92 = dll-call lib="C:/Windows/System32/user32.dll" fn="PostMessageA" label="SendMessageA"("hWnd"=w226, "uMsg"=1130, "wParam"=0, "lParam"=w224) -> ()  [unwired: 8 in, 2 out]
      }
      event Timeout; "Display Cluster Output": Value Change {
        # "button to start to play output cluster"
        n93 = event-data() -> ()  [unwired: 1 in, 2 out]
        n94 = case shown="True" "Display Cluster Output" {
          selector: "Display Cluster Output" -> [_ w243]
          tunnel: w236 -> [_ w249]
          tunnel: w235 -> [_ w248]
          tunnel: w234 -> [_ w247]
          tunnel: w233 -> [_ w246]
          tunnel: w232 -> [_ w242]
          tunnel: w231 -> [_ w241]
          tunnel: w230 -> [_ w240]
          frame False {
          }
          frame True {
            n95 = while {
              tunnel: w249 -> [w263]
              tunnel: w248 -> [w262]
              tunnel: w247 -> [w261]
              tunnel: w246 -> [w260]
              tunnel: [w259] -> w244
              tunnel: [w258] -> w245
              tunnel: w243 -> [w257]
              tunnel: w242 -> [w254]
              tunnel: w241 -> [w253]
              tunnel: w240 -> [w252]
              tunnel: [w251] -> w238
              tunnel: [w250] -> w239
              i -> [w255]
              stop <- w256 stop-if-true
              # "This closes the UDP Multicast connection \nwhen transmission is finished or an error \noccurs"
              # "This closes the UDP connection when\ntransmission is finished or an error occurs"
              n96 = flat-sequence {
                tunnel: w263 -> [w330]
                tunnel: w262 -> [w331]
                tunnel: w261 -> [w332]
                tunnel: w260 -> [w274]
                tunnel: [w329] -> w259
                tunnel: [w328] -> w258
                tunnel: w257 -> [w278]
                tunnel: [w279] -> w256
                tunnel: w255 -> [w285]
                tunnel: w254 -> [w277]
                tunnel: w253 -> [w271]
                tunnel: w252 -> [w276]
                tunnel: [w272] -> w251
                tunnel: [w273] -> w250
                frame #0 {
                  # "This is for testing & hidden"
                  # "This is an input from the VC++.\nThis node is hidden"
                  # "This writes the phasor parameters\ninto a Multicast UDP and send it\nOver LAN and WAN."
                  # "Output cluster that shows the phasor parameter\nin a cluster in \"Output Cluster\" page."
                  # "This writes the phasor parameters\ninto UDP and sends it over LAN, WAN"
                  # "seperate each set of pahsor\nparameters with a \"#\" sign."
                  # "concatenate phasor parameters\nseperated with \";\""
                  # "This part creates index numbers\nto fetch all the phasor parameters\nfor all the time stamps."
                  # "Concatenate Phasor value, timestamp, phasor name, FREQ, DFREQ and\nsend it via unicast UDP connection. here with \"Index of Array of Clusters\" \none can select different parameter values at different time stamps."
                  # "Fetch phasor value, Time Stamp, FREQ, DFREQ from\noutput array. Thus, all the parameters above for a given\ntime stamp are concatenated and send it via unicast UDP\nconnection."
                  # "Write to the Unicast  Address"
                  n97 = local read "output array 4"() -> (w265:string[])
                  "output array 5" <- w265
                  n98 = Re/Im To Complex(1:"Img", 2:"Real") -> (0:w358:cdb[])
                  "Complex Format" <- w358
                  "Complex" <- w358
                  n99 = Insert Into Array(array=w265, index=0, new element="Phasor_Value_Table") -> (w264:string[])
                  n100 = Build Cluster Array(w264, "Phasor Time", "Phasor Values", w358, "DFREQ Values", "FREQ Values") -> (w301:T7)
                  "PDC Output Cluster" <- w301
                  n101 = Index Array "Index Array"(array=w301, index="Index of Array of clusters") -> (element=w356:T8)
                  n102 = Unbundle(w356) -> ("element"=w348:string, "SignalTime"=w344:string, "Numeric"=w351:dbl, "Numeric"=w353:cdb, "Numeric"=w350:dbl, "Numeric"=w349:dbl)
                  "Phasor_Name" <- w348
                  "Rectangular Phasor Values" <- w353
                  "Signal Timestamp" <- w344
                  "Phasor Amplitude/Magnitude" <- w351
                  "DFREQ Value" <- w350
                  "FREQ Value" <- w349
                  n103 = Number To Fractional String(number=w351) -> (F-format string=w341:string)  [unwired: 3 in]
                  n104 = Number To Decimal String(number=w353) -> (decimal integer string=w338:string)  [unwired: 1 in]
                  n105 = Number To Fractional String(number=w350) -> (F-format string=w335:string)  [unwired: 3 in]
                  n106 = Number To Fractional String(number=w349) -> (F-format string=w333:string)  [unwired: 3 in]
                  n107 = Concatenate Strings(w348, ";" ("string")) -> (w346:string)
                  n108 = Concatenate Strings(w344, ";" ("string")) -> (w343:string)
                  n109 = Concatenate Strings(w341, ";" ("string")) -> (w340:string)
                  n110 = Concatenate Strings(w338, ";" ("string")) -> (w337:string)
                  n111 = Concatenate Strings(w335, ";" ("string")) -> (w334:string)
                  n112 = Wait (ms)(milliseconds to wait=u32 100) -> ()  [unwired: 1 out]
                  n113 = Concatenate Strings "Concatenate Strings"(w346, w343, w340, w337, w334, w333) -> ()  [unwired: 1 out]
                  n114 = Array Size(array="Analog Signal") -> (size(s)=w300:i32)
                  n115 = Array Size(array="Digital Signal") -> (size(s)=w284:i32)
                  n116 = Array Size(array=w301) -> (size(s)=w306:i32)
                  n117 = Wait (ms)(milliseconds to wait=u32 100) -> ()  [unwired: 1 out]
                  n118 = Quotient & Remainder(x=w285, y=w306) -> (x-y*floor(x/y)=w270:i32)  [unwired: 1 out]
                  "x-y*floor(x/y)" <- w270
                  n119 = Quotient & Remainder(x=w285, y=w300) -> (x-y*floor(x/y)=w299:i32)  [unwired: 1 out]
                  n120 = Quotient & Remainder(x=w285, y=w284) -> (x-y*floor(x/y)=w290:i32)  [unwired: 1 out]
                  n121 = Index Array "Index Array"(array=w301, index=w270) -> (element=w326:T8)
                  n122 = Index Array "Index Array"(array="Analog Signal", index=w299) -> (element=w296:dbl)
                  n123 = Index Array "Index Array"(array="Digital Signal", index=w290) -> (element=w287:dbl)
                  n124 = Unbundle(w326) -> ("element"=w268:string, "SignalTime"=w311:string, "Numeric"=w310:dbl, "Numeric"=w309:cdb, "Numeric"=w308:dbl, "Numeric"=w307:dbl)
                  n125 = Number To Fractional String(number=w310) -> (F-format string=w320:string)  [unwired: 3 in]
                  n126 = Number To Decimal String(number=w309) -> (decimal integer string=w317:string)  [unwired: 1 in]
                  n127 = Number To Fractional String(number=w308) -> (F-format string=w314:string)  [unwired: 3 in]
                  n128 = Number To Fractional String(number=w307) -> (F-format string=w292:string)  [unwired: 3 in]
                  n129 = Concatenate Strings(w311, ";" ("string")) -> (w322:string)
                  n130 = Number To Fractional String(number=w296) -> (F-format string=w298:string)  [unwired: 3 in]
                  n131 = Number To Fractional String(number=w287) -> (F-format string=w289:string)  [unwired: 3 in]
                  n132 = Concatenate Strings(w268, ";" ("string")) -> (w324:string)
                  n133 = Concatenate Strings(w320, ";" ("string")) -> (w319:string)
                  n134 = Concatenate Strings(w317, ";" ("string")) -> (w316:string)
                  n135 = Concatenate Strings(w314, ";" ("string")) -> (w313:string)
                  n136 = Concatenate Strings(w292, ";" ("string")) -> (w291:string)
                  n137 = Not(x=w278) -> (.not. x?=w303:bool)
                  n138 = Concatenate Strings("Digital String", ";" ("string")) -> (w281:string)
                  n139 = Concatenate Strings(w298, ";" ("string")) -> (w295:string)
                  n140 = Concatenate Strings(w289, ";" ("string")) -> (w283:string)
                  n141 = Concatenate Strings "Concatenate Strings"(w324, w322, w319, w316, w313, w291, w295, w283, w281) -> (w312:string)
                  n142 = Or(x=w303, y="Display Cluster Output 2") -> (x .or. y?=w279:bool)
                  n143 = Concatenate Strings "Entire Data"(w312, "#" ("string")) -> (w275:string)
                  n144 = UDP Write(address=w271, port or service name=w277, connection ID=w276, data in=w275, 8:w274) -> (error out=w272:errorcluster, 3:w273:refnum<k16>)  [unwired: 1 in]
                  n145 = UDP Write(address=w331, port or service name=w330, connection ID=w332, data in=w275, 8:w274) -> (error out=w328:errorcluster, 3:w329:refnum<k16>)  [unwired: 1 in]
                  "Waveform Graph" <- "Phasor Values"
                }
              }
            }
            n146 = UDP Close(connection ID=w244, 8:w245) -> ()  [unwired: 2 out]
            n147 = UDP Close(connection ID=w239, 8:w238) -> ()  [unwired: 2 out]
          }
        }
      }
      event "Save Configuration": Value Change {
        # "This comes from the Chosen data list box\nThis array will be save inthe Write XML file.vi\nas an array for later reference."
        # "Output of the Chosen Data.\nWe will save this in a XML file."
        n148 = event-data() -> ()  [unwired: 1 in, 5 out]
        n149 = case shown="True" "Save Configuration" {
          selector: "Save Configuration" -> [_ w362]
          frame False {
          }
          frame True {
            n150 = flat-sequence {
              tunnel: [w366] -> w363
              tunnel: w362 -> [w374]
              tunnel: w363 -> [w385]
              frame #0 {
                w369 = path "C:/Users/iitc1/Documents" ("start path")
                n151 = call "File Dialog2"("start path"=w369, "default name"="KTHcnf0", "pattern (all files)"="*.xml") -> ("selected path"=w370:path, "cancelled"=w371:bool, "error out"=w372:errorcluster)  [unwired: 9 in, 1 out]
                n152 = Select(t=w369, s=w371, f=w370) -> (s? t:f=w365:path)
                n153 = case shown="True" w374 {
                  tunnel: w365 -> [_ w378]
                  frame False {
                  }
                  frame True {
                    n154 = property class="LstBox (strict)"("Item Names"=string[] []) -> ()  [unwired: 2 in, 2 out]
                    n155 = Open/Create/Replace File(file path (use dialog)=w378, operation (0:open)=T6."replace or create", access (0:read/write)=enum16{"read/write", "read-only", "write-only"}."write-only") -> (error out=w380:errorcluster)  [unwired: 3 in, 2 out]
                    n156 = Open/Create/Replace File(file path (use dialog)=w378, error in=w380) -> (refnum out=w376:refnum<file>, error out=w379:errorcluster)  [unwired: 4 in, 1 out]
                    n157 = Close File(refnum=w376, error in=w379) -> (path=w381:path, error out=w377:errorcluster)
                    n158 = Delete(path (use dialog)=w381, error in=w377) -> (error out=w375:errorcluster)  [unwired: 3 in, 2 out]
                    n159 = call <vilib>:"Clear Errors.vi"("error in (no error)"=w375) -> ()  [unwired: 6 in, 1 out]
                    n160 = call <vilib>:"General Error Handler.vi"() -> ()  [unwired: 11 in, 5 out]
                  }
                }
                n161 = call <vilib>:"Clear Errors.vi"("error in (no error)"=w372) -> ()  [unwired: 6 in, 1 out]
                n162 = Strip Path(path=w365) -> (stripped path=w368:path, name=w367:string)
                n163 = Build Path(base path=w368, name or relative path=w367) -> (appended path=w366:path)
              }
              frame #1 {
                n164 = while {
                  tunnel: w385 -> [w390]
                  i -> [w399]
                  stop <- w397 stop-if-true
                  (unwired) ""
                  n165 = local read "output array 3"() -> (w386:string[])
                  n166 = Array Size(array=w386) -> (size(s)=w398:i32)
                  "size(s)" <- w398
                  n167 = Subtract(x=w398, y=w399) -> (x-y=w391:i32)
                  "x+y" <- w391
                  n168 = Decrement(x=w391) -> (x-1=w392:i32)
                  n169 = Index Array(array=w386, index=w392) -> (element=w389:string)
                  "element 4" <- w389
                  n170 = Flatten To XML(anything=w389) -> (xml string=w395:string)
                  n171 = Equal To 0?(x=w391) -> (x = 0?=w397:bool)
                  n172 = feedback #5() -> (w393:string)  [unwired: 1 in]
                  n173 = call-poly <vilib>:"Write to XML File.vi"("XML Input"=w393, "XML File Path"=w390) -> ("error out"=w387:errorcluster, "XML String"=→"concatenated string":string, "XML File Path(duplicate)"=→"XML File Save Path":path)  [unwired: 7 in]
                  n174 = Concatenate Strings(w395, w393) -> (w394:string)
                  n175 = feedback-in #5(w394) -> ()
                  n176 = call <vilib>:"Clear Errors.vi"("error in (no error)"=w387) -> ()  [unwired: 6 in, 1 out]
                }
              }
            }
          }
        }
      }
      event "Load Configuration": Value Change {
        # "This code opens a a given Config.XML file and reads it and puts it into the Chosen data list box. \nThe objects for opening the xml file and then reading it as an array and inserting it into the list box is chosen\nthere is a mechanism to stop the reading once we get to the end of the xml file. while loop stops once we get \nthere."
        n177 = event-data() -> ()  [unwired: 1 in, 5 out]
        n178 = Not(x=w401) -> (.not. x?=w400:bool)
        n179 = And(x=w400, y=w403) -> (x .and. y?=w402:bool)
        n180 = case shown="True" w402 {
          selector: w402 -> [_ w409]
          tunnel: w404 -> [_ w414]
          tunnel: [0 w413] -> w406
          tunnel: [string[] [] ("Array") w412] -> w405
          frame False {
          }
          frame True {
            n181 = flat-sequence {
              tunnel: w414 -> [w422]
              tunnel: [w422] -> w410
              tunnel: w409 -> [w421]
              tunnel: [w427] -> w413
              tunnel: [w425] -> w412
              tunnel: [w426] -> w411
              tunnel: w410 -> [w428]
              frame #0 {
                n182 = case shown="True" w421 {
                  frame False {
                  }
                  frame True {
                    n183 = property on="Listbox" class="LstBox (strict)"("Item Names"=string[] []) -> ()  [unwired: 2 in, 2 out]
                    n184 = property class="LstBox (strict)"("Item Names"=string[] []) -> ()  [unwired: 2 in, 2 out]
                  }
                }
              }
              frame #1 {
                n185 = while {
                  tunnel: [w441] -> _
                  tunnel: w428 -> [w437]
                  tunnel: [w435] -> w427
                  tunnel: [w431] -> w425
                  tunnel: [w434] -> w426
                  i -> [w435]
                  stop <- w434 stop-if-true
                  n186 = call-poly <vilib>:"Read From XML File.vi"("XML File Path"=w437) -> ("error out"=w429:errorcluster, "XML Elements"=w443:string[], "XML File Path(duplicate)"=→"XML Open File Path":path)  [unwired: 8 in]
                  n187 = Wait (ms)(milliseconds to wait=u32 10) -> ()  [unwired: 1 out]
                  n188 = call <vilib>:"Clear Errors.vi"("error in (no error)"=w429) -> ()  [unwired: 6 in, 1 out]
                  n189 = Array Size(array=w443) -> (size(s)=w438:i32)
                  n190 = Index Array(array=w443, index=w435) -> (element=w440:string)
                  n191 = property on="Listbox" class="LstBox (strict)"() -> ("Item Names"=w432:string[])  [unwired: 2 in, 2 out]
                  n192 = Decrement(x=w438) -> (x-1=w439:i32)
                  n193 = Unflatten From XML(xml string=w440, type=w440) -> (value=w436:string, error out=w441:errorcluster)  [unwired: 1 in]
                  "String" <- w436
                  n194 = Subtract(x=w439, y=w435) -> (x-y=w442:i32)
                  n195 = Insert Into Array(array=w432, index=w435, new element=w436) -> (w431:string[])
                  "Array" <- w431
                  n196 = property on="Listbox" class="LstBox (strict)"("Item Names"=w431) -> ()  [unwired: 2 in, 2 out]
                  n197 = Equal To 0?(x=w442) -> (x = 0?=w434:bool)
                  "Numeric" <- w435
                }
              }
            }
            n198 = case shown="True" w411 {
              frame False {
              }
              frame True {
                n199 = dll-call lib="C:/Windows/System32/user32.dll" fn="FindWindowA"("lpszClassName"=0, "lpszWindowName"="PDC_Process_Dlg" ("lpszWindowName 2")) -> ("return type"=w417:i32)  [unwired: 5 in, 2 out]
                n200 = dll-call lib="C:/Windows/System32/user32.dll" fn="PostMessageA" label="SendMessageA"("hWnd"=w417, "uMsg"=1142, "wParam"=0, "lParam"=0) -> ()  [unwired: 8 in, 2 out]
              }
            }
          }
        }
      }
      event User Event {
        n201 = event-data() -> ("stringMessage"=→"stringMessage":string)  [unwired: 1 in, 3 out]
      }
      event "Analog Parameters": Double Click {
        n202 = event-data() -> ("Row"=w445:i32)  [unwired: 1 in, 7 out]
        n203 = dll-call lib="C:/Windows/System32/user32.dll" fn="FindWindowA"("lpszClassName"=0, "lpszWindowName"="PDC_Process_Dlg" ("lpszWindowName 2")) -> ("return type"=w447:i32)  [unwired: 5 in, 2 out]
        n204 = dll-call lib="C:/Windows/System32/user32.dll" fn="PostMessageA" label="SendMessageA"("hWnd"=w447, "uMsg"=1140, "wParam"=0, "lParam"=w445) -> ()  [unwired: 8 in, 2 out]
      }
      event "Digital Parameters": Double Click {
        n205 = event-data() -> ("Row"=w451:i32)  [unwired: 1 in, 7 out]
        n206 = dll-call lib="C:/Windows/System32/user32.dll" fn="FindWindowA"("lpszClassName"=0, "lpszWindowName"="PDC_Process_Dlg" ("lpszWindowName 2")) -> ("return type"=w453:i32)  [unwired: 5 in, 2 out]
        n207 = dll-call lib="C:/Windows/System32/user32.dll" fn="PostMessageA" label="SendMessageA"("hWnd"=w453, "uMsg"=1141, "wParam"=0, "lParam"=w451) -> ()  [unwired: 8 in, 2 out]
      }
      event Double Click {
        n208 = event-data() -> ("Row"=w457:i32)  [unwired: 1 in, 7 out]
        "Row2" <- w457
        n209 = dll-call lib="C:/Windows/System32/user32.dll" fn="FindWindowA"("lpszClassName"=0, "lpszWindowName"="PDC_Process_Dlg" ("lpszWindowName 3")) -> ("return type"=w459:i32)  [unwired: 5 in, 2 out]
        n210 = dll-call lib="C:/Windows/System32/user32.dll" fn="PostMessageA" label="SendMessageA"("hWnd"=w459, "uMsg"=1133, "wParam"=0, "lParam"=w457) -> ()  [unwired: 8 in, 2 out]
      }
      event "Phasor   Angle": Mouse Down {
        w463 = 0 ("wParam")
        n211 = event-data() -> ()  [unwired: 1 in, 7 out]
        n212 = dll-call lib="C:/Windows/System32/user32.dll" fn="FindWindowA"("lpszClassName"=0, "lpszWindowName"="PDC_Process_Dlg" ("lpszWindowName 4")) -> ("return type"=w464:i32)  [unwired: 5 in, 2 out]
        n213 = dll-call lib="C:/Windows/System32/user32.dll" fn="PostMessageA" label="SendMessageA"("hWnd"=w464, "uMsg"=1130, "wParam"=w463, "lParam"=w463) -> ()  [unwired: 8 in, 2 out]
      }
      event "Quit": Value Change {
        w475 = 0 ("wParam")
        n214 = event-data() -> ("OldVal"=w473:bool, "NewVal"=w472:bool)  [unwired: 1 in, 3 out]
        n215 = Not Equal?(x=w473, y=w472) -> (x != y?=w469:bool)
        n216 = Select(t=0, s=w469, f=2) -> (s? t:f=w468:i32)
        n217 = property on="Save Configuration" class="Bool"("DisabledEnum"=w468) -> ()  [unwired: 2 in, 2 out]
        n218 = dll-call lib="C:/Windows/System32/user32.dll" fn="FindWindowA"("lpszClassName"=0, "lpszWindowName"="PDC_Process_Dlg") -> ("return type"=w474:i32)  [unwired: 5 in, 2 out]
        n219 = property on="Load Configuration" class="Bool (strict)"("DisabledEnum"=w468) -> ()  [unwired: 2 in, 2 out]
        n220 = dll-call lib="C:/Windows/System32/user32.dll" fn="SendMessageA"("hWnd"=w474, "uMsg"=16, "wParam"=w475, "lParam"=w475) -> ()  [unwired: 8 in, 2 out]
      }
      event "Quit 2": Value Change {
        w486 = 0 ("wParam")
        n221 = event-data() -> ("OldVal"=w481:bool, "NewVal"=w480:bool)  [unwired: 1 in, 3 out]
        n222 = Not Equal?(x=w481, y=w480) -> (x != y?=w482:bool)
        n223 = Select(t=0, s=w482, f=2) -> (s? t:f=w479:i32)
        n224 = property on="Save Configuration" class="Bool"("DisabledEnum"=w479) -> ()  [unwired: 2 in, 2 out]
        n225 = property on="Load Configuration" class="Bool (strict)"("DisabledEnum"=w479) -> ()  [unwired: 2 in, 2 out]
        n226 = dll-call lib="C:/Windows/System32/user32.dll" fn="FindWindowA"("lpszClassName"=0, "lpszWindowName"="PDC_Process_Dlg") -> ("return type"=w485:i32)  [unwired: 5 in, 2 out]
        n227 = dll-call lib="C:/Windows/System32/user32.dll" fn="SendMessageA"("hWnd"=w485, "uMsg"=16, "wParam"=w486, "lParam"=w486) -> ()  [unwired: 8 in, 2 out]
      }
      event "Play Chosen Data": Value Change {
        w491 = 0 ("wParam")
        # "This will allow all of the phasor parameters stay\nvisible. in the chose phasor list box when we click\non the play button."
        # "Play button to play chosen data"
        n228 = event-data() -> ("OldVal"=w501:bool, "NewVal"=w500:bool)  [unwired: 1 in, 3 out]
        n229 = Not Equal?(x=w501, y=w500) -> (x != y?=w496:bool)
        n230 = Select(t=2, s=w496, f=0) -> (s? t:f=w497:i32)
        n231 = property on="Save Configuration" class="Bool"("DisabledEnum"=w497) -> ()  [unwired: 2 in, 2 out]
        n232 = property on="Load Configuration" class="Bool (strict)"("DisabledEnum"=w497) -> ()  [unwired: 2 in, 2 out]
        n233 = case shown="True" w495 {
          frame False {
          }
          frame True {
            n234 = property on="Listbox" class="LstBox (strict)"() -> ("Item Names"=w502:string[])  [unwired: 2 in, 2 out]
            n235 = property class="LstBox (strict)"("Item Names"=w502) -> ()  [unwired: 2 in, 2 out]
          }
        }
        n236 = dll-call lib="C:/Windows/System32/user32.dll" fn="FindWindowA"("lpszClassName"=0, "lpszWindowName"="PDC_Process_Dlg") -> ("return type"=w490:i32)  [unwired: 5 in, 2 out]
        n237 = dll-call lib="C:/Windows/System32/user32.dll" fn="SendMessageA"("hWnd"=w490, "uMsg"=1138, "wParam"=w491, "lParam"=w491) -> ()  [unwired: 8 in, 2 out]
      }
      event "stop": Value Change {
        n238 = event-data() -> ()  [unwired: 1 in, 5 out]
      }
      event "A2": Value Change {
        n239 = event-data() -> ("OldVal"=w514:bool[], "NewVal"=w513:bool[])  [unwired: 1 in, 3 out]
        n240 = Not Equal?(x=w514, y=w513) -> (x != y?=w510:bool[])
        n241 = dll-call lib="C:/Windows/System32/user32.dll" fn="FindWindowA"("lpszClassName"=0, "lpszWindowName"="PDC_Process_Dlg" ("lpszWindowName 2")) -> ("return type"=w505:i32)  [unwired: 5 in, 2 out]
        n242 = Search 1D Array(1D array=w510, element=TRUE) -> (index of element=w503:i32)  [unwired: 1 in]
        n243 = Index Array(array=w509, index=w503) -> (element=w511:string)
        n244 = dll-call lib="C:/Windows/System32/user32.dll" fn="PostMessageA" label="SendMessageA"("hWnd"=w505, "uMsg"=1135, "wParam"=0, "lParam"=w503) -> ()  [unwired: 8 in, 2 out]
      }
      event "MA": Value Change {
        n245 = event-data() -> ()  [unwired: 1 in, 5 out]
      }
    }
    "element" <- w171
    "index of element" <- w172
    n246 = Or(x="stop", y=TRUE) -> (x .or. y?=w165:bool)
    n247 = flat-sequence {
      tunnel: ["Send to Port 2"] -> w147
      tunnel: [w188] -> w149
      tunnel: [w177] -> w148
      frame #0 {
        n248 = String To IP(1:"224.0.0.0" ("x")) -> (0:w181:u32)
        n249 = String To IP(1:"Multicast Address 2") -> (0:w177:u32)
        n250 = String To IP(1:"239.255.255.255" ("x")) -> (0:w180:u32)
        n251 = Greater Or Equal?(x=w177, y=w181) -> (x >= y?=w183:bool)
        n252 = Less Or Equal?(x=w177, y=w180) -> (x <= y?=w182:bool)
        n253 = Not And(1:w182, 2:w183) -> (0:w176:bool)
        "Alert Incorrect \nNetwork Info" <- w176
        n254 = case shown="True" w176 {
          frame False {
          }
          frame True {
            n255 = call "Display Message to User2"() -> ()  [unwired: 10 in, 2 out]
          }
        }
        n256 = call-poly <vilib>:"UDP Multicast Open.vi"("time-to-live (1)"="TTL 2", "port"="Local Port 2") -> ("error out"=→"error out":errorcluster, "connection ID"=w188:refnum<k16>)  [unwired: 8 in]
      }
    }
    n257 = And(x="Quit", y=TRUE) -> (x .and. y?=w151:bool)
    n258 = Stop(stop? (T)=w151) -> ()
    n259 = Replace Array Subset(array=w173, new element=w171, index=w172) -> ()  [unwired: 1 out]
    "Quitting" <- "Quit"
  }
  n260 = feedback-in #1(w7) -> ()
  n261 = feedback-in #2(w9) -> ()
  n262 = feedback-in #3(w13) -> ()
  n263 = feedback-in #4(w15) -> ()
  n264 = property class="LstBox (strict)"("Item Names"="PHASORX") -> ()  [unwired: 2 in, 2 out]
  n265 = Index Array(array="PHASORX", index=w21) -> (element=→"Selected Phasor":string)
  n266 = Greater Or Equal To 0?(x=w29) -> (x >= 0?=w33:bool)
  n267 = Select(t=TRUE ("Boolean"), s=w33, f=FALSE) -> (s? t:f=→"bStart":bool)
  n268 = Build Array "Phasor Items"("Phasor Item13", "Phasor Item23", "Phasor Item33", "Phasor Item43") -> ()  [unwired: 1 out]
  n269 = Build Array("output array 2", string[] ["There is no Digital Data"] ("element 2"), string[] ["There is no Frequency Data"] ("element")) -> (w27:string[][])
  n270 = Index Array(array=w27, index (row)=w28) -> (element=w26:string[])  [unwired: 1 in]
  n271 = Build Array "Phasor Items"("Phasor Item102", "Phasor Item202", "Phasor Item302", "Phasor Item402", "Phasor Item502") -> ()  [unwired: 1 out]
  n272 = property class="LstBox (strict)"("Item Names"=w26) -> ()  [unwired: 2 in, 2 out]
  n273 = Build Array "Phasor Items"("Phasor Item1", "Phasor Item2", "Phasor Item3", "Phasor Item4") -> ()  [unwired: 1 out]
  n274 = Build Array "Phasor Items"("Phasor Item12", "Phasor Item22", "Phasor Item32", "Phasor Item42") -> ()  [unwired: 1 out]
  n275 = Build Array "Phasor Items"("Phasor Item14", "Phasor Item24", "Phasor Item34", "Phasor Item44") -> ()  [unwired: 1 out]
